vi "InverseKinematics_4Omni_Trigonon.vi"(0 "VX":dbl, 1 "R_Robot (0.1585m)":dbl=0.1585, 2 "R_Wheel (0.05m)":dbl=0.05, 5 "VY":dbl, 7 "Omega":dbl, 11 "error in (no error)":errorcluster) -> (4 "W1-FL":dbl, 6 "W2-BL":dbl, 8 "W3-FR":dbl, 10 "W4-BR":dbl, 15 "error out":errorcluster)   [LabVIEW 2017]
panel:
  # "Common unit using m/s and rad/s"
  # "Wheel output base on Stupid's Crab wheel position"
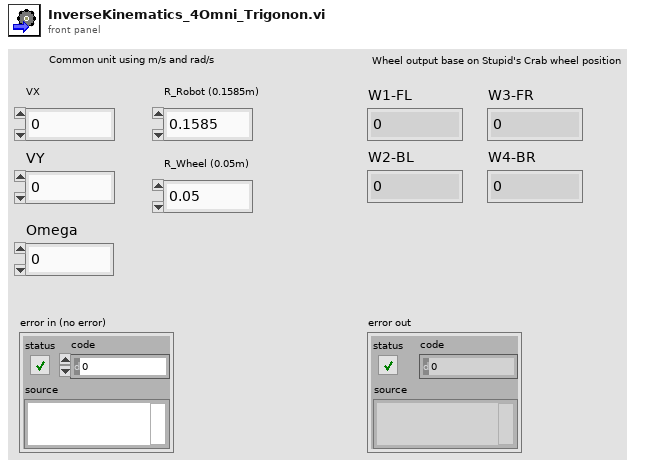
[diagram p1: front panel]
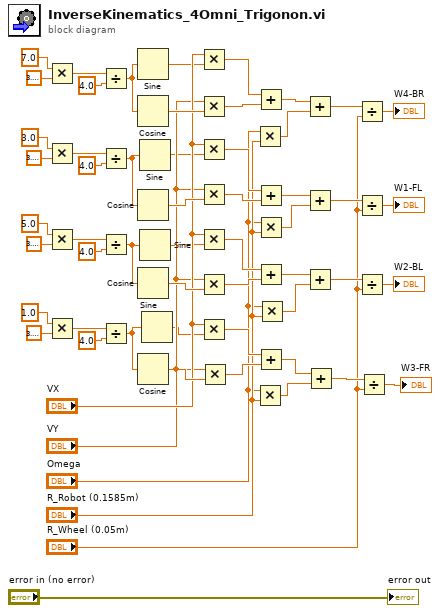
[diagram p0: block diagram]
diagram:
  n1 = Multiply(x=7.0, y=3.141592653589793) -> (x*y=w18:dbl)
  n2 = Multiply(x=3.0, y=3.141592653589793) -> (x*y=w40:dbl)
  n3 = Multiply(x=5.0, y=3.141592653589793) -> (x*y=w29:dbl)
  n4 = Multiply(x=1.0, y=3.141592653589793) -> (x*y=w11:dbl)
  n5 = Divide(x=w18, y=4.0) -> (x/y=w7:dbl)
  n6 = Divide(x=w40, y=4.0) -> (x/y=w2:dbl)
  n7 = Divide(x=w29, y=4.0) -> (x/y=w3:dbl)
  n8 = Divide(x=w11, y=4.0) -> (x/y=w5:dbl)
  n9 = Sine(x=w7) -> (sin(x)=w8:dbl)
  n10 = Cosine(x=w7) -> (cos(x)=w27:dbl)
  n11 = Cosine(x=w2) -> (cos(x)=w49:dbl)
  n12 = Cosine(x=w3) -> (cos(x)=w38:dbl)
  n13 = Cosine(x=w5) -> (cos(x)=w57:dbl)
  n14 = Sine(x=w2) -> (sin(x)=w1:dbl)
  n15 = Sine(x=w3) -> (sin(x)=w4:dbl)
  n16 = Sine(x=w5) -> (sin(x)=w6:dbl)
  n17 = Multiply(x="VX", y=w8) -> (x*y=w25:dbl)
  n18 = Multiply(x="VY", y=w27) -> (x*y=w26:dbl)
  n19 = Multiply(x="VX", y=w1) -> (x*y=w47:dbl)
  n20 = Multiply(x="VY", y=w49) -> (x*y=w48:dbl)
  n21 = Multiply(x="VX", y=w4) -> (x*y=w36:dbl)
  n22 = Multiply(x="VY", y=w38) -> (x*y=w37:dbl)
  n23 = Multiply(x="VX", y=w6) -> (x*y=w55:dbl)
  n24 = Multiply(x="VY", y=w57) -> (x*y=w56:dbl)
  n25 = Multiply(x="Omega", y="R_Robot (0.1585m)") -> (x*y=w23:dbl)
  n26 = Multiply(x="Omega", y="R_Robot (0.1585m)") -> (x*y=w53:dbl)
  n27 = Add(x=w25, y=w26) -> (x+y=w24:dbl)
  n28 = Add(x=w47, y=w48) -> (x+y=w46:dbl)
  n29 = Multiply(x="Omega", y="R_Robot (0.1585m)") -> (x*y=w45:dbl)
  n30 = Add(x=w36, y=w37) -> (x+y=w35:dbl)
  n31 = Add(x=w55, y=w56) -> (x+y=w54:dbl)
  n32 = Multiply(x="Omega", y="R_Robot (0.1585m)") -> (x*y=w34:dbl)
  n33 = Add(x=w24, y=w23) -> (x+y=w22:dbl)
  n34 = Add(x=w46, y=w45) -> (x+y=w44:dbl)
  n35 = Add(x=w35, y=w34) -> (x+y=w33:dbl)
  n36 = Add(x=w54, y=w53) -> (x+y=w52:dbl)
  n37 = Divide(x=w22, y="R_Wheel (0.05m)") -> (x/y=→"W4-BR":dbl)
  n38 = Divide(x=w44, y="R_Wheel (0.05m)") -> (x/y=→"W1-FL":dbl)
  n39 = Divide(x=w33, y="R_Wheel (0.05m)") -> (x/y=→"W2-BL":dbl)
  n40 = Divide(x=w52, y="R_Wheel (0.05m)") -> (x/y=→"W3-FR":dbl)
  "error out" <- "error in (no error)"
